vi "get_number_of_pixels_per_section.vi"(8 "error in (no error)":errorcluster, 11 "TrajectoryDL121017Hopping in":refnum<class "TrajectoryDL121017Hopping.lvclass">) -> (0 "error out":errorcluster, 1 "pixels per uncaging section":i32, 2 "pixels per hopping section":i32, 3 "TrajectoryDL121017Hopping out":refnum<class "TrajectoryDL121017Hopping.lvclass">, 4 "total pixels per section":i32)   [LabVIEW 2010, in "TrajectoryDL121017Hopping.lvclass"]
doc: "Returns the number of pixels per section (there is one section for each ROI):\n\n- for the hopping part of the section\n- for the uncaging part of the section\n- the sum for the two parts."
uses:
  TrajectoryDL121017Hopping.lvclass
  TrajectoryDL121017Hopping.lvclass/TrajectoryDL121017Hopping.ctl
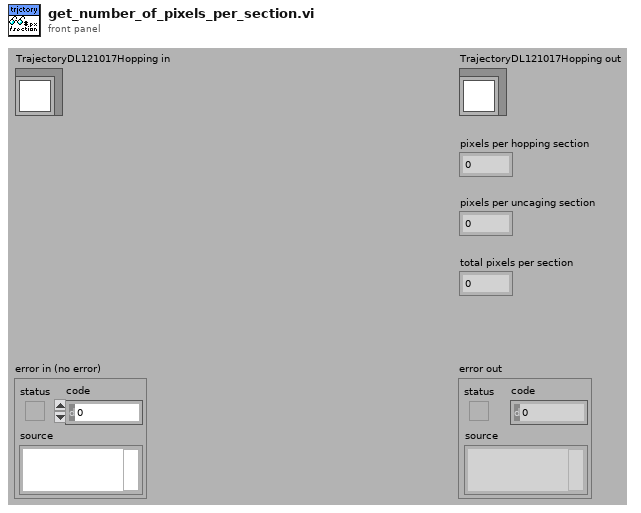
[diagram p1: front panel]
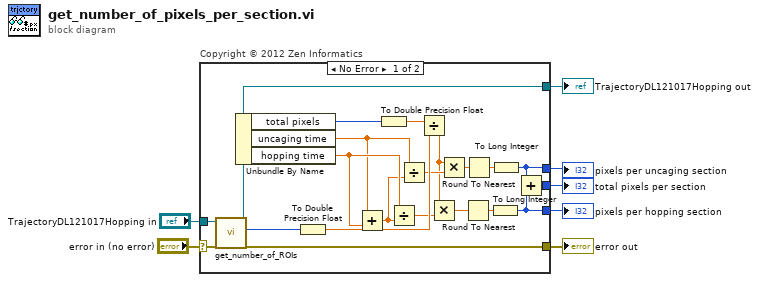
[diagram p0: block diagram]
diagram:
  n1 = case "Copyright © 2012 Zen Informatics" shown="No Error" "error in (no error)" {
    selector: "error in (no error)" -> [w12 w30]
    tunnel: [w11 w30] -> w6
    tunnel: [w8 w29] -> w4
    tunnel: "TrajectoryDL121017Hopping in" -> [w9 w29]
    tunnel: [w15 _] -> w1
    tunnel: [w14 _] -> w2
    tunnel: [w13 _] -> w3
    frame No Error {
      n2 = call "get_number_of_ROIs.vi"("error in (no error)"=w12, "TrajectoryDL121017Hopping in"=w9) -> ("error out"=w11:errorcluster, "number of ROIs"=w10:i32, "TrajectoryDL121017Hopping out"=w8:refnum<class "TrajectoryDL121017Hopping.lvclass">)  [unwired: 7 in]
      n3 = Unbundle By Name(w8) -> ("total pixels"=w26:i32, "uncaging time"=w25:dbl[unit], "hopping time"=w28:dbl[unit])
      n4 = To Double Precision Float(number=w10) -> (double precision float=w22:dbl)
      n5 = Add(x=w25, y=w28) -> (x+y=w24:dbl[unit])
      n6 = To Double Precision Float(number=w26) -> (double precision float=w23:dbl)
      n7 = Divide(x=w28, y=w24) -> (x/y=w21:dbl)
      n8 = Divide(x=w25, y=w24) -> (x/y=w18:dbl)
      n9 = Divide(x=w23, y=w22) -> (x/y=w17:dbl)
      n10 = Multiply(x=w17, y=w21) -> (x*y=w20:dbl)
      n11 = Multiply(x=w17, y=w18) -> (x*y=w16:dbl)
      n12 = Round To Nearest(number=w20) -> (nearest integer value=w27:dbl)
      n13 = Round To Nearest(number=w16) -> (nearest integer value=w19:dbl)
      n14 = To Long Integer(number=w27) -> (32bit integer=w14:i32)
      n15 = To Long Integer(number=w19) -> (32bit integer=w15:i32)
      n16 = Add(x=w15, y=w14) -> (x+y=w13:i32)
    }
    frame Error {
    }
  }
  "error out" <- w6
  "TrajectoryDL121017Hopping out" <- w4
  "pixels per hopping section" <- w2
  "pixels per uncaging section" <- w1
  "total pixels per section" <- w3
